vi "get_[]s.vi"(7 "prefix":string, 11 "String":string) -> (3 "[]Array":string[](array[string]))   [LabVIEW 2022 SP3]
uses:
  <vilib>/Utility/error.llb/Trim Whitespace One-Sided.vi
  <vilib>/regexp/Match Regular Expression.xnode
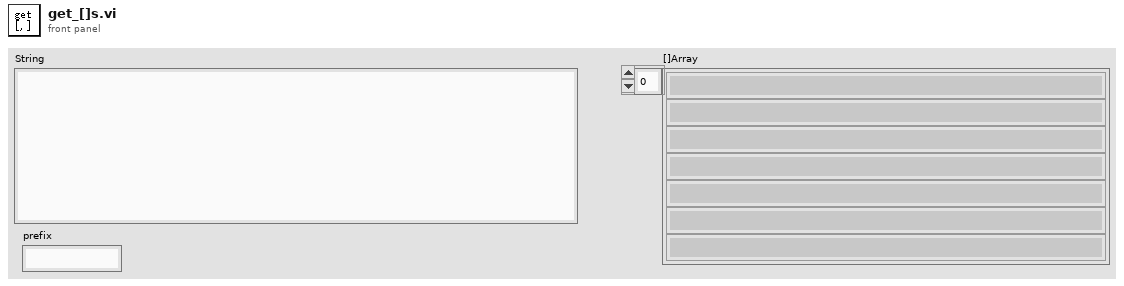
[diagram p1: front panel]
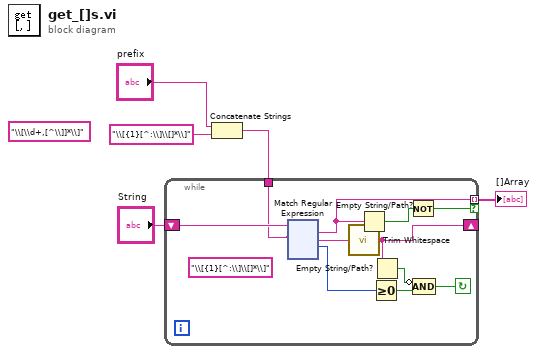
[diagram p0: block diagram]
diagram:
  (unwired) "\\[\\d+,[^\\]]*\\]" ("regular expression")
  n1 = Concatenate Strings("prefix", "\\[{1}[^:\\]\\[]*\\]") -> (w1:string)
  n2 = while {
    shift-right: [w10] -> _
    shift-left: "String" -> [w13]
    tunnel: [w9] -> w5 mode=indexing if=w7
    tunnel: w1 -> [w6]
    stop <- w11 continue-if-true
    (unwired) "\\[{1}[^:\\]\\[]*\\]"
    n3 = xnode "Match Regular Expression"("input string"=w13, "regular expression"=w6) -> ("whole match"=w9:string, "after match"=w15:string, "offset past match"=w12:i32)  [unwired: 4 in, 2 out]
    n4 = call <vilib>:"Trim Whitespace.vi"("string"=w15) -> ("trimmed string"=w10:string)  [unwired: 1 in]
    n5 = Empty String/Path?(string/path=w9) -> (empty?=w8:bool)
    n6 = Greater Or Equal To 0?(x=w12) -> (x >= 0?=w16:bool)
    n7 = Empty String/Path?(string/path=w10) -> (empty?=w14:bool)
    n8 = Not(x=w8) -> (.not. x?=w7:bool)
    n9 = Compound Arithmetic op=AND(invert w14, w16) -> (w11:bool)
  }
  "[]Array" <- w5
